vi "Solve2.vi"(8 "Error In":errorcluster, 11 "object in":refnum<class "2025_2.lvclass">) -> (0 "Error Out":errorcluster, 2 "Result":u64, 3 "object out":refnum<class "2025_2.lvclass">)   [LabVIEW 2025, in "2025_2.lvclass"]
uses:
  2025_2.lvclass
  2025_2.lvclass/2025_2.ctl
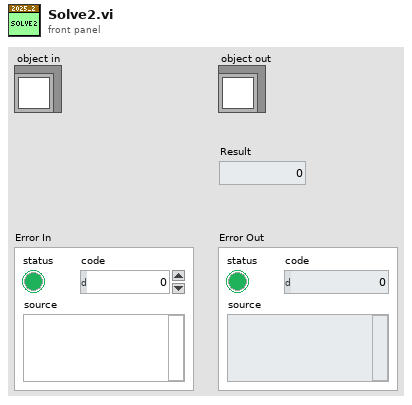
[diagram p1: front panel]
types:
  T1 = typedef "2025_2.lvclass/Range.ctl" = cluster{"Start":u64, "End":u64}
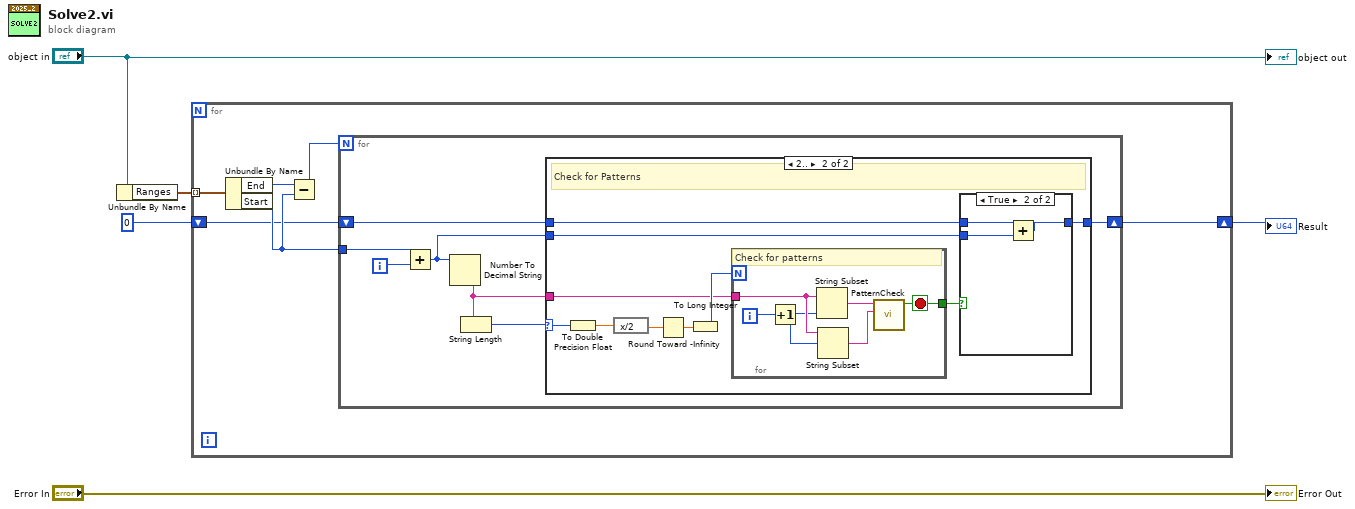
[diagram p0: block diagram]
diagram:
  n1 = Unbundle By Name("object in") -> ("Ranges"=w4:T1[])
  n2 = for {
    tunnel: w4 -> [w11] mode=indexing
    shift-right: [w7] -> w1
    shift-left: u64 0 -> [w6]
    n3 = Unbundle By Name(w11) -> ("End"=w10:u64, "Start"=w8:u64)
    n4 = Subtract(x=w10, y=w8) -> (x-y=w9:u64)
    n5 = for {
      N: w9 -> [_]
      tunnel: w8 -> [w18]
      shift-right: [w14] -> w7
      shift-left: w6 -> [w16]
      i -> [w17]
      n6 = Add(x=w18, y=w17) -> (x+y=w15:u64)
      n7 = Number To Decimal String(number=w15) -> (decimal integer string=w12:string)  [unwired: 1 in]
      n8 = String Length(string=w12) -> (length=w13:i32)
      n9 = case shown="2.." w13 {
        selector: w13 -> [_ w26]
        tunnel: w16 -> [w19 w29]
        tunnel: w15 -> [_ w28]
        tunnel: [w19 w27] -> w14
        tunnel: w12 -> [_ w21]
        frame 0, Default {
        }
        frame 2.. {
          # "Check for Patterns"
          n10 = To Double Precision Float(number=w26) -> (double precision float=w25:dbl)
          n11 = expression code="x/2"(w25) -> (w24:dbl)
          n12 = Round Toward -Infinity(1:w24) -> (0:w23:dbl)
          n13 = To Long Integer(number=w23) -> (32bit integer=w22:i32)
          n14 = for {
            N: w22 -> [_]
            tunnel: w21 -> [w34]
            tunnel: [w30] -> w20
            i -> [w35]
            stop <- w30 stop-if-true
            # "Check for patterns"
            n15 = Increment(x=w35) -> (x+1=w33:i32)
            n16 = String Subset(string=w34, length (rest)=w33) -> (substring=w32:string)  [unwired: 1 in]
            n17 = String Subset(string=w34, offset (0)=w33) -> (substring=w31:string)  [unwired: 1 in]
            n18 = call "PatternCheck.vi"("FullString"=w31, "Pattern 2"=w32) -> ("PatternInString"=w30:bool)  [unwired: 9 in]
          }
          n19 = case shown="True" w20 {
            tunnel: w29 -> [w36 w39]
            tunnel: w28 -> [_ w38]
            tunnel: [w36 w37] -> w27
            frame False {
            }
            frame True {
              n20 = Add(x=w39, y=w38) -> (x+y=w37:u64)
            }
          }
        }
      }
    }
  }
  "Result" <- w1
  "Error Out" <- "Error In"
  "object out" <- "object in"
